vi "Test.vi"() -> ()   [LabVIEW 2020, in "Amium PNS.lvlib"]
uses:
  Amium PNS.lvlib
panel:
  out "Zweites Teil-Array":dbl[](array[numeric])
  out "Erstes Teil-Array":dbl[](array[numeric])
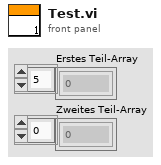
[diagram p1: front panel]
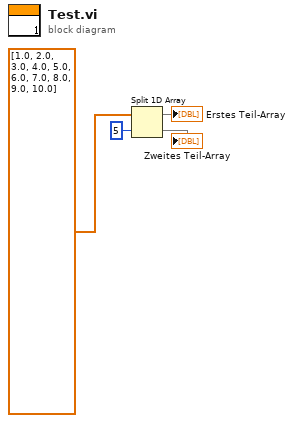
[diagram p0: block diagram]
diagram:
  n1 = Split 1D Array(array=dbl[] [1.0, 2.0, 3.0, 4.0, 5.0, 6.0, 7.0, 8.0, 9.0, 10.0] ("Array"), index=5 ("Index")) -> (first subarray=→"Erstes Teil-Array":dbl[], second subarray=→"Zweites Teil-Array":dbl[])
